vi "NI-DP_RebootDevice.vi"(5 "Port to write to":u16, 6 "Timeout in ms (4s)":u32, 7 "IP to write to":string, 8 "error in (no error)":errorcluster, 9 "MAC Address (hex)":string, 11 "UDP Network Connection in":refnum<k16>) -> (0 "error out":errorcluster, 3 "UDP Network Connection out":refnum<k16>)   [LabVIEW 2014, in "hse-network.lvlib"]
doc: "____\nHAMPEL SOFTWARE ENGINEERING v0.7.0 (2018-07-16 18:12)"
uses:
  hse-network.lvlib
  NI-DP__Commands.ctl
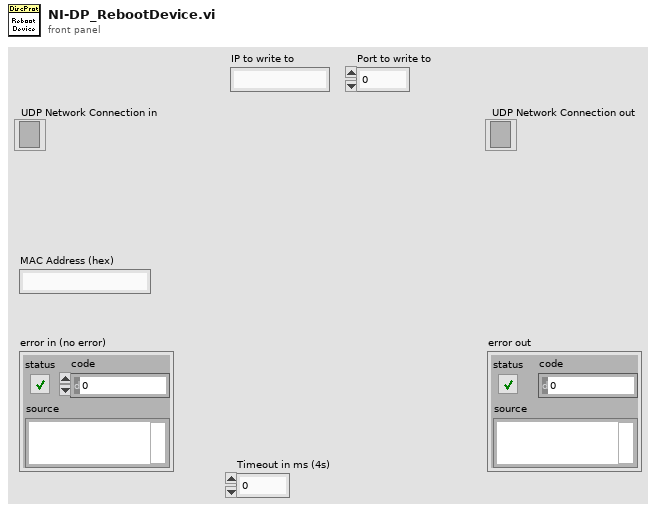
[diagram p1: front panel]
types:
  T1 = typedef "hse-network.lvlib/NI-DP__Commands.ctl" = u8
  T2 = typedef "hse-network.lvlib/NI-DP__MessageStructure.ctl" = cluster{"Start of Message":string, "Command":T1, "Checksum(?) for P3,P4":string, "Always 0x02":string, "Model Code":string, "??? 1":string, "Serial":string, "Device Mac Address":string, "??? 2":string, "Param 1":string, "Param 2":string, "Param 3":string, "Param 4":string, "Checksum(?) for Network":string, "Device IP Address":string, "Device Subnet Mask":string, "Device DNS-Server":string, "Device Default Gateway":string, "??? 3":string, "End of Message":string}
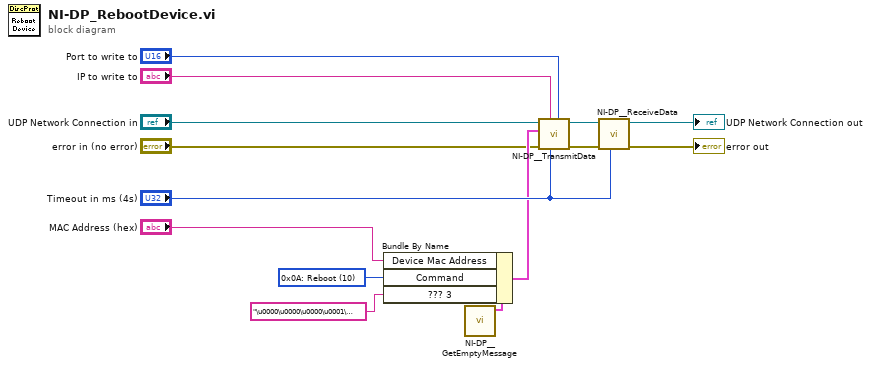
[diagram p0: block diagram]
diagram:
  w10 = T1 10 items=["0x01: Get Type & Hostname"=1, "0x03: Set IP 1"=3, "0x04: Set IP 2"=4, "0x08: Acknowledge"=8, "0x0A: Reboot"=10, "0x20: ???"=32, "0x21: ???"=33, "0xF2: System State"=242, "0xF4: System Details"=244] ("Command")
  n1 = call "NI-DP__GetEmptyMessage.vi"() -> ("NI-DP__EmptyMessage"=w9:T2)  [unwired: 11 in]
  n2 = Bundle By Name(cluster=w9, "Device Mac Address"="MAC Address (hex)", "Command"=w10, "??? 3"="\u0000\u0000\u0000\u0001\u0000\u0000\u0000\u0000") -> (w11:T2)
  n3 = call "NI-DP__TransmitData.vi"("Port to write to"="Port to write to", "timeout ms"="Timeout in ms (4s)", "IP to write to"="IP to write to", "error in"="error in (no error)", "UDP-NI__Message"=w11, "UDP Network Connection in"="UDP Network Connection in") -> ("error out"=w5:errorcluster, "UDP Network Connection out"=w2:refnum<k16>)  [unwired: 4 in]
  n4 = call "NI-DP__ReceiveData.vi"("timeout [ms]"="Timeout in ms (4s)", "error in"=w5, "UDP Network Connection in"=w2) -> ("error out"=→"error out":errorcluster, "UDP Network Connection out"=→"UDP Network Connection out":refnum<k16>)  [unwired: 3 in, 4 out]
